vi "LV to ITX  Retrieve_SE mode.vi"(0 "File or Folder Path":path=path "B:/SketchSET/SA03008H.20180718/51-B+BG_0to15_0.25steps_@0-7T_1step_at.2Hz/SA03008H.20180718.000487.itx", 5 "offset":i32, 7 "length":i32=1, 9 "index":T2={"A"=3, "B"=5, "C"=3, "D"=5, "E"=3, "N1"=2, "N2"=2, "N3"=3, "N4"=4, "A 1"=8, "A 2"=10, "C 1"=5, "C 2"=1, "E 2"=4}, 11 "stop":bool, 12 "file contains 2D data?":bool) -> (1 "Spherical coordinates":dbl[][](array[numeric])=[[9.90056946810301, 45.0, 90.8270537879769]], 2 "long":cluster{i32[], dbl[]}(graph), 3 "G vs T":cluster{dbl[], dbl[]}(graph)={[7.00003046875], [0.0]}, 4 "A vs B":cluster{dbl[], dbl[]}[](graph), 6 "C vs D":cluster{dbl[], dbl[]}[](graph), 8 "E( = A)":dbl[][](graph)=[[0.010896697044372123], [0.010896697044372123], [0.010896697044372123], [0.010896697044372123], [0.010896697044372123], [0.010896697044372123], [0.010896697044372123], [0.010896697044372123], [0.010896697044372123], [0.010896697044372123], [0.010896697044372123], [0.010896697044372123], [0.010896697044372123], [0.010896697044372123], [0.010896697044372123], [0.010896697044372123], [0.010896697044372123], [0.010896697044372123], [0.010896697044372123], [0.010896697044372123], [0.010896697044372123], [0.010896697044372123], [0.010896697044372123], [0.010896697044372123], [0.010896697044372123], [0.010896697044372123], [0.010896697044372123], [0.010896697044372123], [0.010896697044372123], [0.010896697044372123], [0.010896697044372123], [0.010896697044372123], [0.010896697044372123], [0.010896697044372123], [0.010896697044372123], [0.010896697044372123], [0.010896697044372123], [0.010896697044372123], [0.010896697044372123], [0.010896697044372123], [0.010896697044372123], [0.010896697044372123], [0.010896697044372123], [0.010896697044372123], [0.010896697044372123], [0.010896697044372123], [0.010896697044372123], [0.010896697044372123], [0.010896697044372123], [0.010896697044372123], [0.010896697044372123], [0.010896697044372123], [0.010896697044372123], [0.010896697044372123], [0.010896697044372123], [0.010896697044372123], [0.010896697044372123], [0.010896697044372123], [0.010896697044372123], [0.010896697044372123], [0.010896697044372123], [0.010896697044372123], [0.010896697044372123], [0.010896697044372123], [0.010896697044372123], [0.010896697044372123], [0.010896697044372123], [0.010896697044372123], [0.010896697044372123], [0.010896697044372123], [0.010896697044372123], [0.010896697044372123], [0.010896697044372123], [0.010896697044372123], [0.010896697044372123], [0.010896697044372123], [0.010896697044372123], [0.010896697044372123], [0.010896697044372123], [0.010896697044372123], [0.010896697044372123], [0.010896697044372123], [0.010896697044372123], [0.010896697044372123], [0.010896697044372123], [0.010896697044372123], [0.010896697044372123], [0.010896697044372123], [0.010896697044372123], [0.010896697044372123], [0.010896697044372123], [0.010896697044372123], [0.010896697044372123], [0.010896697044372123], [0.010896697044372123], [0.010896697044372123], [0.010896697044372123], [0.010896697044372123], [0.010896697044372123], [0.010896697044372123], [0.010896697044372123], [0.010896697044372123], [0.010896697044372123], [0.010896697044372123], [0.010896697044372123], [0.010896697044372123], [0.010896697044372123], [0.010896697044372123], [0.010896697044372123], [0.010896697044372123], [0.010896697044372123], [0.010896697044372123], [0.010896697044372123], [0.010896697044372123], [0.010896697044372123], [0.010896697044372123], [0.010896697044372123], [0.010896697044372123], [0.010896697044372123], [0.010896697044372123], [0.010896697044372123], [0.010896697044372123], [0.010896697044372123], [0.010896697044372123], [0.010896697044372123], [0.010896697044372123], [0.010896697044372123], [0.010896697044372123], [0.010896697044372123], [0.010896697044372123], [0.010896697044372123], [0.010896697044372123], [0.010896697044372123], [0.010896697044372123], [0.010896697044372123], [0.010896697044372123], [0.010896697044372123], [0.010896697044372123], [0.010896697044372123], [0.010896697044372123], [0.010896697044372123], [0.010896697044372123], [0.010896697044372123], [0.010896697044372123], [0.010896697044372123], [0.010896697044372123], [0.010896697044372123], [0.010896697044372123], [0.010896697044372123], [0.010896697044372123], [0.010896697044372123], [0.010896697044372123], [0.010896697044372123], [0.010896697044372123], [0.010896697044372123], [0.010896697044372123], [0.010896697044372123], [0.010896697044372123], [0.010896697044372123], [0.010896697044372123], [0.010896697044372123], [0.010896697044372123], [0.010896697044372123], [0.010896697044372123], [0.010896697044372123], [0.010896697044372123], [0.010896697044372123], [0.010896697044372123], [0.010896697044372123], [0.010896697044372123], [0.010896697044372123], [0.010896697044372123], [0.010896697044372123], [0.010896697044372123], [0.010896697044372123], [0.010896697044372123], [0.010896697044372123], [0.010896697044372123], [0.010896697044372123], [0.010896697044372123], [0.010896697044372123], [0.010896697044372123], [0.010896697044372123], [0.010896697044372123], [0.010896697044372123], [0.010896697044372123], [0.010896697044372123], [0.010896697044372123], [0.010896697044372123], [0.010896697044372123], [0.010896697044372123], [0.010896697044372123], [0.010896697044372123], [0.010896697044372123], [0.010896697044372123], [0.010896697044372123], [0.010896697044372123], [0.010896697044372123], [0.010896697044372123], [0.010896697044372123], [0.010896697044372123], [0.010896697044372123], [0.010896697044372123], [0.010896697044372123], [0.010896697044372123], [0.010896697044372123], [0.010896697044372123], [0.010896697044372123], [0.010896697044372123], [0.010896697044372123], [0.010896697044372123], [0.010896697044372123], [0.010896697044372123], [0.010896697044372123], [0.010896697044372123], [0.010896697044372123], [0.010896697044372123], [0.010896697044372123], [0.010896697044372123], [0.010896697044372123], [0.010896697044372123], [0.010896697044372123], [0.010896697044372123], [0.010896697044372123], [0.010896697044372123], [0.010896697044372123], [0.010896697044372123], [0.010896697044372123], [0.010896697044372123], [0.010896697044372123], [0.010896697044372123], [0.010896697044372123], [0.010896697044372123], [0.010896697044372123], [0.010896697044372123], [0.010896697044372123], [0.010896697044372123], [0.010896697044372123], [0.010896697044372123], [0.010896697044372123], [0.010896697044372123], [0.010896697044372123], [0.010896697044372123], [0.010896697044372123], [0.010896697044372123], [0.010896697044372123], [0.010896697044372123], [0.010896697044372123], [0.010896697044372123], [0.010896697044372123], [0.010896697044372123], [0.010896697044372123], [0.010896697044372123], [0.010896697044372123], [0.010896697044372123], [0.010896697044372123], [0.010896697044372123], [0.010896697044372123], [0.010896697044372123], [0.010896697044372123], [0.010896697044372123], [0.010896697044372123], [0.010896697044372123], [0.010896697044372123], [0.010896697044372123], [0.010896697044372123], [0.010896697044372123], [0.010896697044372123], [0.010896697044372123], [0.010896697044372123], [0.010896697044372123], [0.010896697044372123], [0.010896697044372123], [0.010896697044372123], [0.010896697044372123], [0.010896697044372123], [0.010896697044372123], [0.010896697044372123], [0.010896697044372123], [0.010896697044372123], [0.010896697044372123], [0.010896697044372123], [0.010896697044372123], [0.010896697044372123], [0.010896697044372123], [0.010896697044372123], [0.010896697044372123], [0.010896697044372123], [0.010896697044372123], [0.010896697044372123], [0.010896697044372123], [0.010896697044372123], [0.010896697044372123], [0.010896697044372123], [0.010896697044372123], [0.010896697044372123], [0.010896697044372123], [0.010896697044372123], [0.010896697044372123], [0.010896697044372123], [0.010896697044372123], [0.010896697044372123], [0.010896697044372123], [0.010896697044372123], [0.010896697044372123], [0.010896697044372123], [0.010896697044372123], [0.010896697044372123], [0.010896697044372123], [0.010896697044372123], [0.010896697044372123], [0.010896697044372123], [0.010896697044372123], [0.010896697044372123], [0.010896697044372123], [0.010896697044372123], [0.010896697044372123], [0.010896697044372123], [0.010896697044372123], [0.010896697044372123], [0.010896697044372123], [0.010896697044372123], [0.010896697044372123], [0.010896697044372123], [0.010896697044372123], [0.010896697044372123], [0.010896697044372123], [0.010896697044372123], [0.010896697044372123], [0.010896697044372123], [0.010896697044372123], [0.010896697044372123], [0.010896697044372123], [0.010896697044372123], [0.010896697044372123], [0.010896697044372123], [0.010896697044372123], [0.010896697044372123], [0.010896697044372123], [0.010896697044372123], [0.010896697044372123], [0.010896697044372123], [0.010896697044372123], [0.010896697044372123], [0.010896697044372123], [0.010896697044372123], [0.010896697044372123], [0.010896697044372123], [0.010896697044372123], [0.010896697044372123], [0.010896697044372123], [0.010896697044372123], [0.010896697044372123], [0.010896697044372123], [0.010896697044372123], [0.010896697044372123], [0.010896697044372123], [0.010896697044372123], [0.010896697044372123], [0.010896697044372123], [0.010896697044372123], [0.010896697044372123], [0.010896697044372123], [0.010896697044372123], [0.010896697044372123], [0.010896697044372123], [0.010896697044372123], [0.010896697044372123], [0.010896697044372123], [0.010896697044372123], [0.010896697044372123], [0.010896697044372123], [0.010896697044372123], [0.010896697044372123], [0.010896697044372123], [0.010896697044372123], [0.010896697044372123], [0.010896697044372123], [0.010896697044372123], [0.010896697044372123], [0.010896697044372123], [0.010896697044372123], [0.010896697044372123], [0.010896697044372123], [0.010896697044372123], [0.010896697044372123], [0.010896697044372123], [0.010896697044372123], [0.010896697044372123], [0.010896697044372123], [0.010896697044372123], [0.010896697044372123], [0.010896697044372123], [0.010896697044372123], [0.010896697044372123], [0.010896697044372123], [0.010896697044372123], [0.010896697044372123], [0.010896697044372123], [0.010896697044372123], [0.010896697044372123], [0.010896697044372123], [0.010896697044372123], [0.010896697044372123], [0.010896697044372123], [0.010896697044372123], [0.010896697044372123], [0.010896697044372123], [0.010896697044372123], [0.010896697044372123], [0.010896697044372123], [0.010896697044372123], [0.010896697044372123], [0.010896697044372123], [0.010896697044372123], [0.010896697044372123], [0.010896697044372123], [0.010896697044372123], [0.010896697044372123], [0.010896697044372123], [0.010896697044372123], [0.010896697044372123], [0.010896697044372123], [0.010896697044372123], [0.010896697044372123], [0.010896697044372123], [0.010896697044372123], [0.010896697044372123], [0.010896697044372123], [0.010896697044372123], [0.010896697044372123], [0.010896697044372123], [0.010896697044372123], [0.010896697044372123], [0.010896697044372123], [0.010896697044372123], [0.010896697044372123], [0.010896697044372123], [0.010896697044372123], [0.010896697044372123], [0.010896697044372123], [0.010896697044372123], [0.010896697044372123], [0.010896697044372123], [0.010896697044372123], [0.010896697044372123], [0.010896697044372123], [0.010896697044372123], [0.010896697044372123], [0.010896697044372123], [0.010896697044372123], [0.010896697044372123], [0.010896697044372123], [0.010896697044372123], [0.010896697044372123], [0.010896697044372123], [0.010896697044372123], [0.010896697044372123], [0.010896697044372123], [0.010896697044372123], [0.010896697044372123], [0.010896697044372123], [0.010896697044372123], [0.010896697044372123], [0.010896697044372123], [0.010896697044372123], [0.010896697044372123], [0.010896697044372123], [0.010896697044372123], [0.010896697044372123], [0.010896697044372123], [0.010896697044372123], [0.010896697044372123], [0.010896697044372123], [0.010896697044372123], [0.010896697044372123], [0.010896697044372123], [0.010896697044372123], [0.010896697044372123], [0.010896697044372123], [0.010896697044372123], [0.010896697044372123], [0.010896697044372123], [0.010896697044372123], [0.010896697044372123], [0.010896697044372123], [0.010896697044372123], [0.010896697044372123], [0.010896697044372123], [0.010896697044372123], [0.010896697044372123], [0.010896697044372123], [0.010896697044372123], [0.010896697044372123], [0.010896697044372123], [0.010896697044372123], [0.010896697044372123], [0.010896697044372123], [0.010896697044372123], [0.010896697044372123], [0.010896697044372123], [0.010896697044372123], [0.010896697044372123], [0.010896697044372123], [0.010896697044372123], [0.010896697044372123], [0.010896697044372123], [0.010896697044372123], [0.010896697044372123], [0.010896697044372123], [0.010896697044372123], [0.010896697044372123], [0.010896697044372123], [0.010896697044372123], [0.010896697044372123], [0.010896697044372123], [0.010896697044372123], [0.010896697044372123], [0.010896697044372123], [0.010896697044372123], [0.010896697044372123], [0.010896697044372123], [0.010896697044372123], [0.010896697044372123], [0.010896697044372123], [0.010896697044372123], [0.010896697044372123], [0.010896697044372123], [0.010896697044372123], [0.010896697044372123], [0.010896697044372123], [0.010896697044372123], [0.010896697044372123], [0.010896697044372123], [0.010896697044372123], [0.010896697044372123], [0.010896697044372123], [0.010896697044372123], [0.010896697044372123], [0.010896697044372123], [0.010896697044372123], [0.010896697044372123], [0.010896697044372123], [0.010896697044372123], [0.010896697044372123], [0.010896697044372123], [0.010896697044372123], [0.010896697044372123], [0.010896697044372123], [0.010896697044372123], [0.010896697044372123], [0.010896697044372123], [0.010896697044372123], [0.010896697044372123], [0.010896697044372123], [0.010896697044372123], [0.010896697044372123], [0.010896697044372123], [0.010896697044372123], [0.010896697044372123], [0.010896697044372123], [0.010896697044372123], [0.010896697044372123], [0.010896697044372123], [0.010896697044372123], [0.010896697044372123], [0.010896697044372123], [0.010896697044372123], [0.010896697044372123], [0.010896697044372123], [0.010896697044372123], [0.010896697044372123], [0.010896697044372123], [0.010896697044372123], [0.010896697044372123], [0.010896697044372123], [0.010896697044372123], [0.010896697044372123], [0.010896697044372123], [0.010896697044372123], [0.010896697044372123], [0.010896697044372123], [0.010896697044372123], [0.010896697044372123], [0.010896697044372123], [0.010896697044372123], [0.010896697044372123], [0.010896697044372123], [0.010896697044372123], [0.010896697044372123], [0.010896697044372123], [0.010896697044372123], [0.010896697044372123], [0.010896697044372123], [0.010896697044372123], [0.010896697044372123], [0.010896697044372123], [0.010896697044372123], [0.010896697044372123], [0.010896697044372123], [0.010896697044372123], [0.010896697044372123], [0.010896697044372123], [0.010896697044372123], [0.010896697044372123], [0.010896697044372123], [0.010896697044372123], [0.010896697044372123], [0.010896697044372123], [0.010896697044372123], [0.010896697044372123], [0.010896697044372123], [0.010896697044372123], [0.010896697044372123], [0.010896697044372123], [0.010896697044372123], [0.010896697044372123], [0.010896697044372123], [0.010896697044372123], [0.010896697044372123], [0.010896697044372123], [0.010896697044372123], [0.010896697044372123], [0.010896697044372123], [0.010896697044372123], [0.010896697044372123], [0.010896697044372123], [0.010896697044372123], [0.010896697044372123], [0.010896697044372123], [0.010896697044372123], [0.010896697044372123], [0.010896697044372123], [0.010896697044372123], [0.010896697044372123], [0.010896697044372123], [0.010896697044372123], [0.010896697044372123], [0.010896697044372123], [0.010896697044372123], [0.010896697044372123], [0.010896697044372123], [0.010896697044372123], [0.010896697044372123], [0.010896697044372123], [0.010896697044372123], [0.010896697044372123], [0.010896697044372123], [0.010896697044372123], [0.010896697044372123], [0.010896697044372123], [0.010896697044372123], [0.010896697044372123], [0.010896697044372123], [0.010896697044372123], [0.010896697044372123], [0.010896697044372123], [0.010896697044372123], [0.010896697044372123], [0.010896697044372123], [0.010896697044372123], [0.010896697044372123], [0.010896697044372123], [0.010896697044372123], [0.010896697044372123], [0.010896697044372123], [0.010896697044372123], [0.010896697044372123], [0.010896697044372123], [0.010896697044372123], [0.010896697044372123], [0.010896697044372123], [0.010896697044372123], [0.010896697044372123], [0.010896697044372123], [0.010896697044372123], [0.010896697044372123], [0.010896697044372123], [0.010896697044372123], [0.010896697044372123], [0.010896697044372123], [0.010896697044372123], [0.010896697044372123], [0.010896697044372123], [0.010896697044372123], [0.010896697044372123], [0.010896697044372123], [0.010896697044372123], [0.010896697044372123], [0.010896697044372123], [0.010896697044372123], [0.010896697044372123], [0.010896697044372123], [0.010896697044372123], [0.010896697044372123], [0.010896697044372123], [0.010896697044372123], [0.010896697044372123], [0.010896697044372123], [0.010896697044372123], [0.010896697044372123], [0.010896697044372123], [0.010896697044372123], [0.010896697044372123], [0.010896697044372123], [0.010896697044372123], [0.010896697044372123], [0.010896697044372123], [0.010896697044372123], [0.010896697044372123], [0.010896697044372123], [0.010896697044372123], [0.010896697044372123], [0.010896697044372123], [0.010896697044372123], [0.010896697044372123], [0.010896697044372123], [0.010896697044372123], [0.010896697044372123], [0.010896697044372123], [0.010896697044372123], [0.010896697044372123], [0.010896697044372123], [0.010896697044372123], [0.010896697044372123], [0.010896697044372123], [0.010896697044372123], [0.010896697044372123], [0.010896697044372123], [0.010896697044372123], [0.010896697044372123], [0.010896697044372123], [0.010896697044372123], [0.010896697044372123], [0.010896697044372123], [0.010896697044372123], [0.010896697044372123], [0.010896697044372123], [0.010896697044372123], [0.010896697044372123], [0.010896697044372123], [0.010896697044372123], [0.010896697044372123], [0.010896697044372123], [0.010896697044372123], [0.010896697044372123], [0.010896697044372123], [0.010896697044372123], [0.010896697044372123], [0.010896697044372123], [0.010896697044372123], [0.010896697044372123], [0.010896697044372123], [0.010896697044372123], [0.010896697044372123], [0.010896697044372123], [0.010896697044372123], [0.010896697044372123], [0.010896697044372123], [0.010896697044372123], [0.010896697044372123], [0.010896697044372123], [0.010896697044372123], [0.010896697044372123], [0.010896697044372123], [0.010896697044372123], [0.010896697044372123], [0.010896697044372123], [0.010896697044372123], [0.010896697044372123], [0.010896697044372123], [0.010896697044372123], [0.010896697044372123], [0.010896697044372123], [0.010896697044372123], [0.010896697044372123], [0.010896697044372123], [0.010896697044372123], [0.010896697044372123], [0.010896697044372123], [0.010896697044372123], [0.010896697044372123], [0.010896697044372123], [0.010896697044372123], [0.010896697044372123], [0.010896697044372123], [0.010896697044372123], [0.010896697044372123], [0.010896697044372123], [0.010896697044372123], [0.010896697044372123], [0.010896697044372123], [0.010896697044372123], [0.010896697044372123], [0.010896697044372123], [0.010896697044372123], [0.010896697044372123], [0.010896697044372123], [0.010896697044372123], [0.010896697044372123], [0.010896697044372123], [0.010896697044372123], [0.010896697044372123], [0.010896697044372123], [0.010896697044372123], [0.010896697044372123], [0.010896697044372123], [0.010896697044372123], [0.010896697044372123], [0.010896697044372123], [0.010896697044372123], [0.010896697044372123], [0.010896697044372123], [0.010896697044372123], [0.010896697044372123], [0.010896697044372123], [0.010896697044372123], [0.010896697044372123], [0.010896697044372123], [0.010896697044372123], [0.010896697044372123], [0.010896697044372123], [0.010896697044372123], [0.010896697044372123], [0.010896697044372123], [0.010896697044372123], [0.010896697044372123], [0.010896697044372123], [0.010896697044372123], [0.010896697044372123], [0.010896697044372123], [0.010896697044372123], [0.010896697044372123], [0.010896697044372123], [0.010896697044372123], [0.010896697044372123], [0.010896697044372123], [0.010896697044372123], [0.010896697044372123], [0.010896697044372123], [0.010896697044372123], [0.010896697044372123], [0.010896697044372123], [0.010896697044372123], [0.010896697044372123], [0.010896697044372123], [0.010896697044372123], [0.010896697044372123], [0.010896697044372123], [0.010896697044372123], [0.010896697044372123], [0.010896697044372123], [0.010896697044372123], [0.010896697044372123], [0.010896697044372123], [0.010896697044372123], [0.010896697044372123], [0.010896697044372123], [0.010896697044372123], [0.010896697044372123], [0.010896697044372123], [0.010896697044372123], [0.010896697044372123], [0.010896697044372123], [0.010896697044372123], [0.010896697044372123], [0.010896697044372123], [0.010896697044372123], [0.010896697044372123], [0.010896697044372123], [0.010896697044372123], [0.010896697044372123], [0.010896697044372123], [0.010896697044372123], [0.010896697044372123], [0.010896697044372123], [0.010896697044372123], [0.010896697044372123], [0.010896697044372123], [0.010896697044372123], [0.010896697044372123], [0.010896697044372123], [0.010896697044372123], [0.010896697044372123], [0.010896697044372123], [0.010896697044372123], [0.010896697044372123], [0.010896697044372123], [0.010896697044372123], [0.010896697044372123], [0.010896697044372123], [0.010896697044372123], [0.010896697044372123], [0.010896697044372123], [0.010896697044372123], [0.010896697044372123], [0.010896697044372123], [0.010896697044372123], [0.010896697044372123], [0.010896697044372123], [0.010896697044372123], [0.010896697044372123], [0.010896697044372123], [0.010896697044372123], [0.010896697044372123], [0.010896697044372123], [0.010896697044372123], [0.010896697044372123], [0.010896697044372123], [0.010896697044372123], [0.010896697044372123], [0.010896697044372123], [0.010896697044372123], [0.010896697044372123], [0.010896697044372123], [0.010896697044372123], [0.010896697044372123], [0.010896697044372123], [0.010896697044372123], [0.010896697044372123], [0.010896697044372123], [0.010896697044372123], [0.010896697044372123], [0.010896697044372123], [0.010896697044372123], [0.010896697044372123], [0.010896697044372123], [0.010896697044372123], [0.010896697044372123], [0.010896697044372123], [0.010896697044372123], [0.010896697044372123], [0.010896697044372123], [0.010896697044372123], [0.010896697044372123], [0.010896697044372123], [0.010896697044372123], [0.010896697044372123], [0.010896697044372123], [0.010896697044372123], [0.010896697044372123], [0.010896697044372123], [0.010896697044372123], [0.010896697044372123], [0.010896697044372123], [0.010896697044372123], [0.010896697044372123], [0.010896697044372123], [0.010896697044372123], [0.010896697044372123], [0.010896697044372123], [0.010896697044372123], [0.010896697044372123], [0.010896697044372123], [0.010896697044372123], [0.010896697044372123], [0.010896697044372123], [0.010896697044372123], [0.010896697044372123], [0.010896697044372123], [0.010896697044372123], [0.010896697044372123], [0.010896697044372123], [0.010896697044372123], [0.010896697044372123], [0.010896697044372123], [0.010896697044372123], [0.010896697044372123], [0.010896697044372123], [0.010896697044372123], [0.010896697044372123], [0.010896697044372123], [0.010896697044372123], [0.010896697044372123], [0.010896697044372123], [0.010896697044372123], [0.010896697044372123], [0.010896697044372123], [0.010896697044372123], [0.010896697044372123], [0.010896697044372123], [0.010896697044372123], [0.010896697044372123], [0.010896697044372123], [0.010896697044372123], [0.010896697044372123], [0.010896697044372123], [0.010896697044372123], [0.010896697044372123], [0.010896697044372123], [0.010896697044372123], [0.010896697044372123], [0.010896697044372123], [0.010896697044372123], [0.010896697044372123], [0.010896697044372123], [0.010896697044372123], [0.010896697044372123], [0.010896697044372123], [0.010896697044372123], [0.010896697044372123], [0.010896697044372123], [0.010896697044372123], [0.010896697044372123], [0.010896697044372123], [0.010896697044372123], [0.010896697044372123], [0.010896697044372123], [0.010896697044372123], [0.010896697044372123], [0.010896697044372123], [0.010896697044372123], [0.010896697044372123], [0.010896697044372123], [0.010896697044372123], [0.010896697044372123], [0.010896697044372123], [0.010896697044372123], [0.010896697044372123], [0.010896697044372123], [0.010896697044372123], [0.010896697044372123], [0.010896697044372123], [0.010896697044372123], [0.010896697044372123], [0.010896697044372123], [0.010896697044372123], [0.010896697044372123], [0.010896697044372123], [0.010896697044372123], [0.010896697044372123], [0.010896697044372123], [0.010896697044372123], [0.010896697044372123], [0.010896697044372123], [0.010896697044372123], [0.010896697044372123], [0.010896697044372123], [0.010896697044372123], [0.010896697044372123], [0.010896697044372123], [0.010896697044372123], [0.010896697044372123], [0.010896697044372123], [0.010896697044372123], [0.010896697044372123], [0.010896697044372123], [0.010896697044372123], [0.010896697044372123], [0.010896697044372123], [0.010896697044372123], [0.010896697044372123], [0.010896697044372123], [0.010896697044372123], [0.010896697044372123], [0.010896697044372123], [0.010896697044372123], [0.010896697044372123], [0.010896697044372123], [0.010896697044372123], [0.010896697044372123], [0.010896697044372123], [0.010896697044372123], [0.010896697044372123], [0.010896697044372123], [0.010896697044372123], [0.010896697044372123], [0.010896697044372123], [0.010896697044372123], [0.010896697044372123], [0.010896697044372123], [0.010896697044372123], [0.010896697044372123], [0.010896697044372123], [0.010896697044372123], [0.010896697044372123], [0.010896697044372123], [0.010896697044372123], [0.010896697044372123], [0.010896697044372123], [0.010896697044372123], [0.010896697044372123], [0.010896697044372123], [0.010896697044372123], [0.010896697044372123], [0.010896697044372123], [0.010896697044372123], [0.010896697044372123], [0.010896697044372123], [0.010896697044372123], [0.010896697044372123], [0.010896697044372123], [0.010896697044372123], [0.010896697044372123], [0.010896697044372123], [0.010896697044372123], [0.010896697044372123], [0.010896697044372123], [0.010896697044372123], [0.010896697044372123], [0.010896697044372123], [0.010896697044372123], [0.010896697044372123], [0.010896697044372123], [0.010896697044372123], [0.010896697044372123], [0.010896697044372123], [0.010896697044372123], [0.010896697044372123], [0.010896697044372123], [0.010896697044372123], [0.010896697044372123], [0.010896697044372123], [0.010896697044372123], [0.010896697044372123], [0.010896697044372123], [0.010896697044372123], [0.010896697044372123], [0.010896697044372123], [0.010896697044372123], [0.010896697044372123], [0.010896697044372123], [0.010896697044372123], [0.010896697044372123], [0.010896697044372123], [0.010896697044372123], [0.010896697044372123], [0.010896697044372123], [0.010896697044372123], [0.010896697044372123], [0.010896697044372123], [0.010896697044372123], [0.010896697044372123], [0.010896697044372123], [0.010896697044372123], [0.010896697044372123], [0.010896697044372123], [0.010896697044372123], [0.010896697044372123], [0.010896697044372123], [0.010896697044372123], [0.010896697044372123], [0.010896697044372123], [0.010896697044372123], [0.010896697044372123], [0.010896697044372123], [0.010896697044372123], [0.010896697044372123], [0.010896697044372123], [0.010896697044372123], [0.010896697044372123], [0.010896697044372123], [0.010896697044372123], [0.010896697044372123], [0.010896697044372123], [0.010896697044372123], [0.010896697044372123], [0.010896697044372123], [0.010896697044372123], [0.010896697044372123], [0.010896697044372123], [0.010896697044372123], [0.010896697044372123], [0.010896697044372123], [0.010896697044372123], [0.010896697044372123], [0.010896697044372123], [0.010896697044372123], [0.010896697044372123], [0.010896697044372123], [0.010896697044372123], [0.010896697044372123], [0.010896697044372123], [0.010896697044372123], [0.010896697044372123], [0.010896697044372123], [0.010896697044372123], [0.010896697044372123], [0.010896697044372123], [0.010896697044372123], [0.010896697044372123], [0.010896697044372123], [0.010896697044372123], [0.010896697044372123], [0.010896697044372123], [0.010896697044372123], [0.010896697044372123], [0.010896697044372123], [0.010896697044372123], [0.010896697044372123], [0.010896697044372123], [0.010896697044372123], [0.010896697044372123], [0.010896697044372123], [0.010896697044372123], [0.010896697044372123], [0.010896697044372123], [0.010896697044372123], [0.010896697044372123], [0.010896697044372123], [0.010896697044372123], [0.010896697044372123], [0.010896697044372123], [0.010896697044372123], [0.010896697044372123], [0.010896697044372123], [0.010896697044372123], [0.010896697044372123], [0.010896697044372123], [0.010896697044372123], [0.010896697044372123], [0.010896697044372123], [0.010896697044372123], [0.010896697044372123], [0.010896697044372123], [0.010896697044372123], [0.010896697044372123], [0.010896697044372123], [0.010896697044372123], [0.010896697044372123], [0.010896697044372123], [0.010896697044372123], [0.010896697044372123], [0.010896697044372123], [0.010896697044372123], [0.010896697044372123], [0.010896697044372123], [0.010896697044372123], [0.010896697044372123], [0.010896697044372123], [0.010896697044372123], [0.010896697044372123], [0.010896697044372123], [0.010896697044372123], [0.010896697044372123], [0.010896697044372123], [0.010896697044372123], [0.010896697044372123], [0.010896697044372123], [0.010896697044372123], [0.010896697044372123], [0.010896697044372123], [0.010896697044372123], [0.010896697044372123], [0.010896697044372123], [0.010896697044372123], [0.010896697044372123], [0.010896697044372123], [0.010896697044372123], [0.010896697044372123], [0.010896697044372123], [0.010896697044372123], [0.010896697044372123], [0.010896697044372123], [0.010896697044372123], [0.010896697044372123], [0.010896697044372123], [0.010896697044372123], [0.010896697044372123], [0.010896697044372123], [0.010896697044372123], [0.010896697044372123], [0.010896697044372123], [0.010896697044372123], [0.010896697044372123], [0.010896697044372123], [0.010896697044372123], [0.010896697044372123], [0.010896697044372123], [0.010896697044372123], [0.010896697044372123], [0.010896697044372123], [0.010896697044372123], [0.010896697044372123], [0.010896697044372123], [0.010896697044372123], [0.010896697044372123], [0.010896697044372123], [0.010896697044372123], [0.010896697044372123], [0.010896697044372123], [0.010896697044372123], [0.010896697044372123], [0.010896697044372123], [0.010896697044372123], [0.010896697044372123], [0.010896697044372123], [0.010896697044372123], [0.010896697044372123], [0.010896697044372123], [0.010896697044372123], [0.010896697044372123], [0.010896697044372123], [0.010896697044372123], [0.010896697044372123], [0.010896697044372123], [0.010896697044372123], [0.010896697044372123], [0.010896697044372123], [0.010896697044372123], [0.010896697044372123], [0.010896697044372123], [0.010896697044372123], [0.010896697044372123], [0.010896697044372123], [0.010896697044372123], [0.010896697044372123], [0.010896697044372123], [0.010896697044372123], [0.010896697044372123], [0.010896697044372123], [0.010896697044372123], [0.010896697044372123], [0.010896697044372123], [0.010896697044372123], [0.010896697044372123], [0.010896697044372123], [0.010896697044372123], [0.010896697044372123], [0.010896697044372123], [0.010896697044372123], [0.010896697044372123], [0.010896697044372123], [0.010896697044372123], [0.010896697044372123], [0.010896697044372123], [0.010896697044372123], [0.010896697044372123], [0.010896697044372123], [0.010896697044372123], [0.010896697044372123], [0.010896697044372123], [0.010896697044372123], [0.010896697044372123], [0.010896697044372123], [0.010896697044372123], [0.010896697044372123], [0.010896697044372123], [0.010896697044372123], [0.010896697044372123], [0.010896697044372123], [0.010896697044372123], [0.010896697044372123], [0.010896697044372123], [0.010896697044372123], [0.010896697044372123], [0.010896697044372123], [0.010896697044372123], [0.010896697044372123], [0.010896697044372123], [0.010896697044372123], [0.010896697044372123], [0.010896697044372123], [0.010896697044372123], [0.010896697044372123], [0.010896697044372123], [0.010896697044372123], [0.010896697044372123], [0.010896697044372123], [0.010896697044372123], [0.010896697044372123], [0.010896697044372123], [0.010896697044372123], [0.010896697044372123], [0.010896697044372123], [0.010896697044372123], [0.010896697044372123], [0.010896697044372123], [0.010896697044372123], [0.010896697044372123], [0.010896697044372123], [0.010896697044372123], [0.010896697044372123], [0.010896697044372123], [0.010896697044372123], [0.010896697044372123], [0.010896697044372123], [0.010896697044372123], [0.010896697044372123], [0.010896697044372123], [0.010896697044372123], [0.010896697044372123], [0.010896697044372123], [0.010896697044372123], [0.010896697044372123], [0.010896697044372123], [0.010896697044372123], [0.010896697044372123], [0.010896697044372123], [0.010896697044372123], [0.010896697044372123], [0.010896697044372123], [0.010896697044372123], [0.010896697044372123], [0.010896697044372123], [0.010896697044372123], [0.010896697044372123], [0.010896697044372123], [0.010896697044372123], [0.010896697044372123], [0.010896697044372123], [0.010896697044372123], [0.010896697044372123], [0.010896697044372123], [0.010896697044372123], [0.010896697044372123], [0.010896697044372123], [0.010896697044372123], [0.010896697044372123], [0.010896697044372123], [0.010896697044372123], [0.010896697044372123], [0.010896697044372123], [0.010896697044372123], [0.010896697044372123], [0.010896697044372123], [0.010896697044372123], [0.010896697044372123], [0.010896697044372123], [0.010896697044372123], [0.010896697044372123], [0.010896697044372123], [0.010896697044372123], [0.010896697044372123], [0.010896697044372123], [0.010896697044372123], [0.010896697044372123], [0.010896697044372123], [0.010896697044372123], [0.010896697044372123], [0.010896697044372123], [0.010896697044372123], [0.010896697044372123], [0.010896697044372123], [0.010896697044372123], [0.010896697044372123], [0.010896697044372123], [0.010896697044372123], [0.010896697044372123], [0.010896697044372123], [0.010896697044372123], [0.010896697044372123], [0.010896697044372123], [0.010896697044372123], [0.010896697044372123], [0.010896697044372123], [0.010896697044372123], [0.010896697044372123], [0.010896697044372123], [0.010896697044372123], [0.010896697044372123], [0.010896697044372123], [0.010896697044372123], [0.010896697044372123], [0.010896697044372123], [0.010896697044372123], [0.010896697044372123], [0.010896697044372123], [0.010896697044372123], [0.010896697044372123], [0.010896697044372123], [0.010896697044372123], [0.010896697044372123], [0.010896697044372123], [0.010896697044372123], [0.010896697044372123], [0.010896697044372123], [0.010896697044372123], [0.010896697044372123], [0.010896697044372123], [0.010896697044372123], [0.010896697044372123], [0.010896697044372123], [0.010896697044372123], [0.010896697044372123], [0.010896697044372123], [0.010896697044372123], [0.010896697044372123], [0.010896697044372123], [0.010896697044372123], [0.010896697044372123], [0.010896697044372123], [0.010896697044372123], [0.010896697044372123], [0.010896697044372123], [0.010896697044372123], [0.010896697044372123], [0.010896697044372123], [0.010896697044372123], [0.010896697044372123], [0.010896697044372123], [0.010896697044372123], [0.010896697044372123], [0.010896697044372123], [0.010896697044372123], [0.010896697044372123], [0.010896697044372123], [0.010896697044372123], [0.010896697044372123], [0.010896697044372123], [0.010896697044372123], [0.010896697044372123], [0.010896697044372123], [0.010896697044372123], [0.010896697044372123], [0.010896697044372123], [0.010896697044372123], [0.010896697044372123], [0.010896697044372123], [0.010896697044372123], [0.010896697044372123], [0.010896697044372123], [0.010896697044372123], [0.010896697044372123], [0.010896697044372123], [0.010896697044372123], [0.010896697044372123], [0.010896697044372123], [0.010896697044372123], [0.010896697044372123], [0.010896697044372123], [0.010896697044372123], [0.010896697044372123], [0.010896697044372123], [0.010896697044372123], [0.010896697044372123], [0.010896697044372123], [0.010896697044372123], [0.010896697044372123], [0.010896697044372123], [0.010896697044372123], [0.010896697044372123], [0.010896697044372123], [0.010896697044372123], [0.010896697044372123], [0.010896697044372123], [0.010896697044372123], [0.010896697044372123], [0.010896697044372123], [0.010896697044372123], [0.010896697044372123], [0.010896697044372123], [0.010896697044372123], [0.010896697044372123], [0.010896697044372123], [0.010896697044372123], [0.010896697044372123], [0.010896697044372123], [0.010896697044372123], [0.010896697044372123], [0.010896697044372123], [0.010896697044372123], [0.010896697044372123], [0.010896697044372123], [0.010896697044372123], [0.010896697044372123], [0.010896697044372123], [0.010896697044372123], [0.010896697044372123], [0.010896697044372123], [0.010896697044372123], [0.010896697044372123], [0.010896697044372123], [0.010896697044372123], [0.010896697044372123], [0.010896697044372123], [0.010896697044372123], [0.010896697044372123], [0.010896697044372123], [0.010896697044372123], [0.010896697044372123], [0.010896697044372123], [0.010896697044372123], [0.010896697044372123], [0.010896697044372123], [0.010896697044372123], [0.010896697044372123], [0.010896697044372123], [0.010896697044372123], [0.010896697044372123], [0.010896697044372123], [0.010896697044372123], [0.010896697044372123], [0.010896697044372123], [0.010896697044372123], [0.010896697044372123], [0.010896697044372123], [0.010896697044372123], [0.010896697044372123], [0.010896697044372123], [0.010896697044372123], [0.010896697044372123], [0.010896697044372123], [0.010896697044372123], [0.010896697044372123], [0.010896697044372123], [0.010896697044372123], [0.010896697044372123], [0.010896697044372123], [0.010896697044372123], [0.010896697044372123], [0.010896697044372123], [0.010896697044372123], [0.010896697044372123], [0.010896697044372123], [0.010896697044372123], [0.010896697044372123], [0.010896697044372123], [0.010896697044372123], [0.010896697044372123], [0.010896697044372123], [0.010896697044372123], [0.010896697044372123], [0.010896697044372123], [0.010896697044372123], [0.010896697044372123], [0.010896697044372123], [0.010896697044372123], [0.010896697044372123], [0.010896697044372123], [0.010896697044372123], [0.010896697044372123], [0.010896697044372123], [0.010896697044372123], [0.010896697044372123], [0.010896697044372123], [0.010896697044372123], [0.010896697044372123], [0.010896697044372123], [0.010896697044372123], [0.010896697044372123], [0.010896697044372123], [0.010896697044372123], [0.010896697044372123], [0.010896697044372123], [0.010896697044372123], [0.010896697044372123], [0.010896697044372123], [0.010896697044372123], [0.010896697044372123], [0.010896697044372123], [0.010896697044372123], [0.010896697044372123], [0.010896697044372123], [0.010896697044372123], [0.010896697044372123], [0.010896697044372123], [0.010896697044372123], [0.010896697044372123], [0.010896697044372123], [0.010896697044372123], [0.010896697044372123], [0.010896697044372123], [0.010896697044372123], [0.010896697044372123], [0.010896697044372123], [0.010896697044372123], [0.010896697044372123], [0.010896697044372123], [0.010896697044372123], [0.010896697044372123], [0.010896697044372123], [0.010896697044372123], [0.010896697044372123], [0.010896697044372123], [0.010896697044372123], [0.010896697044372123], [0.010896697044372123], [0.010896697044372123], [0.010896697044372123], [0.010896697044372123], [0.010896697044372123], [0.010896697044372123], [0.010896697044372123], [0.010896697044372123], [0.010896697044372123], [0.010896697044372123], [0.010896697044372123], [0.010896697044372123], [0.010896697044372123], [0.010896697044372123], [0.010896697044372123], [0.010896697044372123], [0.010896697044372123], [0.010896697044372123], [0.010896697044372123], [0.010896697044372123], [0.010896697044372123], [0.010896697044372123], [0.010896697044372123], [0.010896697044372123], [0.010896697044372123], [0.010896697044372123], [0.010896697044372123], [0.010896697044372123], [0.010896697044372123], [0.010896697044372123], [0.010896697044372123], [0.010896697044372123], [0.010896697044372123], [0.010896697044372123], [0.010896697044372123], [0.010896697044372123], [0.010896697044372123], [0.010896697044372123], [0.010896697044372123], [0.010896697044372123], [0.010896697044372123], [0.010896697044372123], [0.010896697044372123], [0.010896697044372123], [0.010896697044372123], [0.010896697044372123], [0.010896697044372123], [0.010896697044372123], [0.010896697044372123], [0.010896697044372123], [0.010896697044372123], [0.010896697044372123], [0.010896697044372123], [0.010896697044372123], [0.010896697044372123], [0.010896697044372123], [0.010896697044372123], [0.010896697044372123], [0.010896697044372123], [0.010896697044372123], [0.010896697044372123], [0.010896697044372123], [0.010896697044372123], [0.010896697044372123], [0.010896697044372123], [0.010896697044372123], [0.010896697044372123], [0.010896697044372123], [0.010896697044372123], [0.010896697044372123], [0.010896697044372123], [0.010896697044372123], [0.010896697044372123], [0.010896697044372123], [0.010896697044372123], [0.010896697044372123], [0.010896697044372123], [0.010896697044372123], [0.010896697044372123], [0.010896697044372123], [0.010896697044372123], [0.010896697044372123], [0.010896697044372123], [0.010896697044372123], [0.010896697044372123], [0.010896697044372123], [0.010896697044372123], [0.010896697044372123], [0.010896697044372123], [0.010896697044372123], [0.010896697044372123], [0.010896697044372123], [0.010896697044372123], [0.010896697044372123], [0.010896697044372123], [0.010896697044372123], [0.010896697044372123], [0.010896697044372123], [0.010896697044372123], [0.010896697044372123], [0.010896697044372123], [0.010896697044372123], [0.010896697044372123], [0.010896697044372123], [0.010896697044372123], [0.010896697044372123], [0.010896697044372123], [0.010896697044372123], [0.010896697044372123], [0.010896697044372123], [0.010896697044372123], [0.010896697044372123], [0.010896697044372123], [0.010896697044372123], [0.010896697044372123], [0.010896697044372123], [0.010896697044372123], [0.010896697044372123], [0.010896697044372123], [0.010896697044372123], [0.010896697044372123], [0.010896697044372123], [0.010896697044372123], [0.010896697044372123], [0.010896697044372123], [0.010896697044372123], [0.010896697044372123], [0.010896697044372123], [0.010896697044372123], [0.010896697044372123], [0.010896697044372123], [0.010896697044372123], [0.010896697044372123], [0.010896697044372123], [0.010896697044372123], [0.010896697044372123], [0.010896697044372123], [0.010896697044372123], [0.010896697044372123], [0.010896697044372123], [0.010896697044372123], [0.010896697044372123], [0.010896697044372123], [0.010896697044372123], [0.010896697044372123], [0.010896697044372123], [0.010896697044372123], [0.010896697044372123], [0.010896697044372123], [0.010896697044372123], [0.010896697044372123], [0.010896697044372123], [0.010896697044372123], [0.010896697044372123], [0.010896697044372123], [0.010896697044372123], [0.010896697044372123], [0.010896697044372123], [0.010896697044372123], [0.010896697044372123], [0.010896697044372123], [0.010896697044372123], [0.010896697044372123], [0.010896697044372123], [0.010896697044372123], [0.010896697044372123], [0.010896697044372123], [0.010896697044372123], [0.010896697044372123], [0.010896697044372123], [0.010896697044372123], [0.010896697044372123], [0.010896697044372123], [0.010896697044372123], [0.010896697044372123], [0.010896697044372123], [0.010896697044372123], [0.010896697044372123], [0.010896697044372123], [0.010896697044372123], [0.010896697044372123], [0.010896697044372123], [0.010896697044372123], [0.010896697044372123], [0.010896697044372123], [0.010896697044372123], [0.010896697044372123], [0.010896697044372123], [0.010896697044372123], [0.010896697044372123], [0.010896697044372123], [0.010896697044372123], [0.010896697044372123], [0.010896697044372123], [0.010896697044372123], [0.010896697044372123], [0.010896697044372123], [0.010896697044372123], [0.010896697044372123], [0.010896697044372123], [0.010896697044372123], [0.010896697044372123], [0.010896697044372123], [0.010896697044372123], [0.010896697044372123], [0.010896697044372123], [0.010896697044372123], [0.010896697044372123], [0.010896697044372123], [0.010896697044372123], [0.010896697044372123], [0.010896697044372123], [0.010896697044372123], [0.010896697044372123], [0.010896697044372123], [0.010896697044372123], [0.010896697044372123], [0.010896697044372123], [0.010896697044372123], [0.010896697044372123], [0.010896697044372123], [0.010896697044372123], [0.010896697044372123], [0.010896697044372123], [0.010896697044372123], [0.010896697044372123], [0.010896697044372123], [0.010896697044372123], [0.010896697044372123], [0.010896697044372123], [0.010896697044372123], [0.010896697044372123], [0.010896697044372123], [0.010896697044372123], [0.010896697044372123], [0.010896697044372123], [0.010896697044372123], [0.010896697044372123], [0.010896697044372123], [0.010896697044372123], [0.010896697044372123], [0.010896697044372123], [0.010896697044372123], [0.010896697044372123], [0.010896697044372123], [0.010896697044372123], [0.010896697044372123], [0.010896697044372123], [0.010896697044372123], [0.010896697044372123], [0.010896697044372123], [0.010896697044372123], [0.010896697044372123], [0.010896697044372123], [0.010896697044372123], [0.010896697044372123], [0.010896697044372123], [0.010896697044372123], [0.010896697044372123], [0.010896697044372123], [0.010896697044372123], [0.010896697044372123], [0.010896697044372123], [0.010896697044372123], [0.010896697044372123], [0.010896697044372123], [0.010896697044372123], [0.010896697044372123], [0.010896697044372123], [0.010896697044372123], [0.010896697044372123], [0.010896697044372123], [0.010896697044372123], [0.010896697044372123], [0.010896697044372123], [0.010896697044372123], [0.010896697044372123], [0.010896697044372123], [0.010896697044372123], [0.010896697044372123], [0.010896697044372123], [0.010896697044372123], [0.010896697044372123], [0.010896697044372123], [0.010896697044372123], [0.010896697044372123], [0.010896697044372123], [0.010896697044372123], [0.010896697044372123], [0.010896697044372123], [0.010896697044372123], [0.010896697044372123], [0.010896697044372123], [0.010896697044372123], [0.010896697044372123], [0.010896697044372123], [0.010896697044372123], [0.010896697044372123], [0.010896697044372123], [0.010896697044372123], [0.010896697044372123], [0.010896697044372123], [0.010896697044372123], [0.010896697044372123], [0.010896697044372123], [0.010896697044372123], [0.010896697044372123], [0.010896697044372123], [0.010896697044372123], [0.010896697044372123], [0.010896697044372123], [0.010896697044372123], [0.010896697044372123], [0.010896697044372123], [0.010896697044372123], [0.010896697044372123], [0.010896697044372123], [0.010896697044372123], [0.010896697044372123], [0.010896697044372123], [0.010896697044372123], [0.010896697044372123], [0.010896697044372123], [0.010896697044372123], [0.010896697044372123], [0.010896697044372123], [0.010896697044372123], [0.010896697044372123], [0.010896697044372123], [0.010896697044372123], [0.010896697044372123], [0.010896697044372123], [0.010896697044372123], [0.010896697044372123], [0.010896697044372123], [0.010896697044372123], [0.010896697044372123], [0.010896697044372123], [0.010896697044372123], [0.010896697044372123], [0.010896697044372123], [0.010896697044372123], [0.010896697044372123], [0.010896697044372123], [0.010896697044372123], [0.010896697044372123], [0.010896697044372123], [0.010896697044372123], [0.010896697044372123], [0.010896697044372123], [0.010896697044372123], [0.010896697044372123], [0.010896697044372123], [0.010896697044372123], [0.010896697044372123], [0.010896697044372123], [0.010896697044372123], [0.010896697044372123], [0.010896697044372123], [0.010896697044372123], [0.010896697044372123], [0.010896697044372123], [0.010896697044372123], [0.010896697044372123], [0.010896697044372123], [0.010896697044372123], [0.010896697044372123], [0.010896697044372123], [0.010896697044372123], [0.010896697044372123], [0.010896697044372123], [0.010896697044372123], [0.010896697044372123], [0.010896697044372123], [0.010896697044372123], [0.010896697044372123], [0.010896697044372123], [0.010896697044372123], [0.010896697044372123], [0.010896697044372123], [0.010896697044372123], [0.010896697044372123], [0.010896697044372123], [0.010896697044372123], [0.010896697044372123], [0.010896697044372123], [0.010896697044372123], [0.010896697044372123], [0.010896697044372123], [0.010896697044372123], [0.010896697044372123], [0.010896697044372123], [0.010896697044372123], [0.010896697044372123], [0.010896697044372123], [0.010896697044372123], [0.010896697044372123], [0.010896697044372123], [0.010896697044372123], [0.010896697044372123], [0.010896697044372123], [0.010896697044372123], [0.010896697044372123], [0.010896697044372123], [0.010896697044372123], [0.010896697044372123], [0.010896697044372123], [0.010896697044372123], [0.010896697044372123], [0.010896697044372123], [0.010896697044372123], [0.010896697044372123], [0.010896697044372123], [0.010896697044372123], [0.010896697044372123], [0.010896697044372123], [0.010896697044372123], [0.010896697044372123], [0.010896697044372123], [0.010896697044372123], [0.010896697044372123], [0.010896697044372123], [0.010896697044372123], [0.010896697044372123], [0.010896697044372123], [0.010896697044372123], [0.010896697044372123], [0.010896697044372123], [0.010896697044372123], [0.010896697044372123], [0.010896697044372123], [0.010896697044372123], [0.010896697044372123], [0.010896697044372123], [0.010896697044372123], [0.010896697044372123], [0.010896697044372123], [0.010896697044372123], [0.010896697044372123], [0.010896697044372123], [0.010896697044372123], [0.010896697044372123], [0.010896697044372123], [0.010896697044372123], [0.010896697044372123], [0.010896697044372123], [0.010896697044372123], [0.010896697044372123], [0.010896697044372123], [0.010896697044372123], [0.010896697044372123], [0.010896697044372123], [0.010896697044372123], [0.010896697044372123], [0.010896697044372123], [0.010896697044372123], [0.010896697044372123], [0.010896697044372123], [0.010896697044372123], [0.010896697044372123], [0.010896697044372123], [0.010896697044372123], [0.010896697044372123], [0.010896697044372123], [0.010896697044372123], [0.010896697044372123], [0.010896697044372123], [0.010896697044372123], [0.010896697044372123], [0.010896697044372123], [0.010896697044372123], [0.010896697044372123], [0.010896697044372123], [0.010896697044372123], [0.010896697044372123], [0.010896697044372123], [0.010896697044372123], [0.010896697044372123], [0.010896697044372123], [0.010896697044372123], [0.010896697044372123], [0.010896697044372123], [0.010896697044372123], [0.010896697044372123], [0.010896697044372123], [0.010896697044372123], [0.010896697044372123], [0.010896697044372123], [0.010896697044372123], [0.010896697044372123], [0.010896697044372123], [0.010896697044372123], [0.010896697044372123], [0.010896697044372123], [0.010896697044372123], [0.010896697044372123], [0.010896697044372123], [0.010896697044372123], [0.010896697044372123], [0.010896697044372123], [0.010896697044372123], [0.010896697044372123], [0.010896697044372123], [0.010896697044372123], [0.010896697044372123], [0.010896697044372123], [0.010896697044372123], [0.010896697044372123], [0.010896697044372123], [0.010896697044372123], [0.010896697044372123], [0.010896697044372123], [0.010896697044372123], [0.010896697044372123], [0.010896697044372123], [0.010896697044372123], [0.010896697044372123], [0.010896697044372123], [0.010896697044372123], [0.010896697044372123], [0.010896697044372123], [0.010896697044372123], [0.010896697044372123], [0.010896697044372123], [0.010896697044372123], [0.010896697044372123], [0.010896697044372123], [0.010896697044372123], [0.010896697044372123], [0.010896697044372123], [0.010896697044372123], [0.010896697044372123], [0.010896697044372123], [0.010896697044372123], [0.010896697044372123], [0.010896697044372123], [0.010896697044372123], [0.010896697044372123], [0.010896697044372123], [0.010896697044372123], [0.010896697044372123], [0.010896697044372123], [0.010896697044372123], [0.010896697044372123], [0.010896697044372123], [0.010896697044372123], [0.010896697044372123], [0.010896697044372123], [0.010896697044372123], [0.010896697044372123], [0.010896697044372123], [0.010896697044372123], [0.010896697044372123], [0.010896697044372123], [0.010896697044372123], [0.010896697044372123], [0.010896697044372123], [0.010896697044372123], [0.010896697044372123], [0.010896697044372123], [0.010896697044372123], [0.010896697044372123], [0.010896697044372123], [0.010896697044372123], [0.010896697044372123], [0.010896697044372123], [0.010896697044372123], [0.010896697044372123], [0.010896697044372123], [0.010896697044372123], [0.010896697044372123], [0.010896697044372123], [0.010896697044372123], [0.010896697044372123], [0.010896697044372123], [0.010896697044372123], [0.010896697044372123], [0.010896697044372123], [0.010896697044372123], [0.010896697044372123], [0.010896697044372123], [0.010896697044372123], [0.010896697044372123], [0.010896697044372123], [0.010896697044372123], [0.010896697044372123], [0.010896697044372123], [0.010896697044372123], [0.010896697044372123], [0.010896697044372123], [0.010896697044372123], [0.010896697044372123], [0.010896697044372123], [0.010896697044372123], [0.010896697044372123], [0.010896697044372123], [0.010896697044372123], [0.010896697044372123], [0.010896697044372123], [0.010896697044372123], [0.010896697044372123], [0.010896697044372123], [0.010896697044372123], [0.010896697044372123], [0.010896697044372123], [0.010896697044372123], [0.010896697044372123], [0.010896697044372123], [0.010896697044372123], [0.010896697044372123], [0.010896697044372123], [0.010896697044372123], [0.010896697044372123], [0.010896697044372123], [0.010896697044372123], [0.010896697044372123], [0.010896697044372123], [0.010896697044372123], [0.010896697044372123], [0.010896697044372123], [0.010896697044372123], [0.010896697044372123], [0.010896697044372123], [0.010896697044372123], [0.010896697044372123], [0.010896697044372123], [0.010896697044372123], [0.010896697044372123], [0.010896697044372123], [0.010896697044372123], [0.010896697044372123], [0.010896697044372123], [0.010896697044372123], [0.010896697044372123], [0.010896697044372123], [0.010896697044372123], [0.010896697044372123], [0.010896697044372123], [0.010896697044372123], [0.010896697044372123], [0.010896697044372123], [0.010896697044372123], [0.010896697044372123], [0.010896697044372123], [0.010896697044372123], [0.010896697044372123], [0.010896697044372123], [0.010896697044372123], [0.010896697044372123], [0.010896697044372123], [0.010896697044372123], [0.010896697044372123], [0.010896697044372123], [0.010896697044372123], [0.010896697044372123], [0.010896697044372123], [0.010896697044372123], [0.010896697044372123], [0.010896697044372123], [0.010896697044372123], [0.010896697044372123], [0.010896697044372123], [0.010896697044372123], [0.010896697044372123], [0.010896697044372123], [0.010896697044372123], [0.010896697044372123], [0.010896697044372123], [0.010896697044372123], [0.010896697044372123], [0.010896697044372123], [0.010896697044372123], [0.010896697044372123], [0.010896697044372123], [0.010896697044372123], [0.010896697044372123], [0.010896697044372123], [0.010896697044372123], [0.010896697044372123], [0.010896697044372123], [0.010896697044372123], [0.010896697044372123], [0.010896697044372123], [0.010896697044372123], [0.010896697044372123], [0.010896697044372123], [0.010896697044372123], [0.010896697044372123], [0.010896697044372123], [0.010896697044372123], [0.010896697044372123], [0.010896697044372123], [0.010896697044372123], [0.010896697044372123], [0.010896697044372123], [0.010896697044372123], [0.010896697044372123], [0.010896697044372123], [0.010896697044372123], [0.010896697044372123], [0.010896697044372123], [0.010896697044372123], [0.010896697044372123], [0.010896697044372123], [0.010896697044372123], [0.010896697044372123], [0.010896697044372123], [0.010896697044372123], [0.010896697044372123], [0.010896697044372123], [0.010896697044372123], [0.010896697044372123], [0.010896697044372123], [0.010896697044372123], [0.010896697044372123], [0.010896697044372123], [0.010896697044372123], [0.010896697044372123], [0.010896697044372123], [0.010896697044372123], [0.010896697044372123], [0.010896697044372123], [0.010896697044372123], [0.010896697044372123], [0.010896697044372123], [0.010896697044372123], [0.010896697044372123], [0.010896697044372123], [0.010896697044372123], [0.010896697044372123], [0.010896697044372123], [0.010896697044372123], [0.010896697044372123], [0.010896697044372123], [0.010896697044372123], [0.010896697044372123], [0.010896697044372123], [0.010896697044372123], [0.010896697044372123], [0.010896697044372123], [0.010896697044372123], [0.010896697044372123], [0.010896697044372123], [0.010896697044372123], [0.010896697044372123], [0.010896697044372123], [0.010896697044372123], [0.010896697044372123], [0.010896697044372123], [0.010896697044372123], [0.010896697044372123], [0.010896697044372123], [0.010896697044372123], [0.010896697044372123], [0.010896697044372123], [0.010896697044372123], [0.010896697044372123], [0.010896697044372123], [0.010896697044372123], [0.010896697044372123], [0.010896697044372123], [0.010896697044372123], [0.010896697044372123], [0.010896697044372123], [0.010896697044372123], [0.010896697044372123], [0.010896697044372123], [0.010896697044372123], [0.010896697044372123], [0.010896697044372123], [0.010896697044372123], [0.010896697044372123], [0.010896697044372123], [0.010896697044372123], [0.010896697044372123], [0.010896697044372123], [0.010896697044372123], [0.010896697044372123], [0.010896697044372123], [0.010896697044372123], [0.010896697044372123], [0.010896697044372123], [0.010896697044372123], [0.010896697044372123], [0.010896697044372123], [0.010896697044372123], [0.010896697044372123], [0.010896697044372123], [0.010896697044372123], [0.010896697044372123], [0.010896697044372123], [0.010896697044372123], [0.010896697044372123], [0.010896697044372123], [0.010896697044372123], [0.010896697044372123], [0.010896697044372123], [0.010896697044372123], [0.010896697044372123], [0.010896697044372123], [0.010896697044372123], [0.010896697044372123], [0.010896697044372123], [0.010896697044372123], [0.010896697044372123], [0.010896697044372123], [0.010896697044372123], [0.010896697044372123], [0.010896697044372123], [0.010896697044372123], [0.010896697044372123], [0.010896697044372123], [0.010896697044372123], [0.010896697044372123], [0.010896697044372123], [0.010896697044372123], [0.010896697044372123], [0.010896697044372123], [0.010896697044372123], [0.010896697044372123], [0.010896697044372123], [0.010896697044372123], [0.010896697044372123], [0.010896697044372123], [0.010896697044372123], [0.010896697044372123], [0.010896697044372123], [0.010896697044372123], [0.010896697044372123], [0.010896697044372123], [0.010896697044372123], [0.010896697044372123], [0.010896697044372123]], 10 "N":cluster{"N1":dbl, "N2":dbl, "N3":dbl, "N4":dbl}={"N1"=7.00003046875, "N2"=7.00003046875, "N3"=-0.14290789298293544, "N4"=-9.432270749714217e-10} {"N4" format="%#_6p"; "N3" format="%#_6p"; "N2" format="%#_6p"; "N1" format="%#_6p"}, 13 "Index, Wavenames":string[][](table)=[["0", "'time.SA03008H.20180718.000487'\n"], ["1", "'temp.SA03008H.20180718.000487'\n"], ["2", "'B.SA03008H.20180718.000487'\n"], ["3", "'Vsource.SA03008H.20180718.000487'\n"], ["4", "'Lockin0.SA03008H.20180718.000487'\n"], ["5", "'Lockin1.SA03008H.20180718.000487'\n"], ["6", "'Lockin2.SA03008H.20180718.000487'\n"], ["7", "'Lockin3.SA03008H.20180718.000487'\n"], ["8", "'Lockin4.SA03008H.20180718.000487'\n"], ["9", "'Lockin5.SA03008H.20180718.000487'\n"], ["10", "'B_rate.SA03008H.20180718.000487'\n"], ["11", "'DC0.SA03008H.20180718.000487'\n"], ["12", "'DC1.SA03008H.20180718.000487'\n"], ["13", "'DC2.SA03008H.20180718.000487'\n"], ["14", "'DC3.SA03008H.20180718.000487'\n"], ["15", "'DC4.SA03008H.20180718.000487'\n"], ["16", "'DC5.SA03008H.20180718.000487'\n"], ["17", "'DC6.SA03008H.20180718.000487'\n"], ["18", "'DC7.SA03008H.20180718.000487'\n"], ["", ""]], 14 "Comments":string="IGOR\nX// Date: 7/19/2018 6:19 PM\nX// SA03008H\nX// \nX// Source 2 Drain 28 (lockin 1 and 7)\nX// Gohm resistor, sweep BG\nX// \nX// 50mV AC -150mV DC for the IV sweep\nX// \nX// 0 to 15 slowly at 0.25 V step sizes\nX// Stepping B 0-7 @ 1T steps\n\nX// B_Field=7.000000\n\nX// \n\nX// B_Field_Rate=0.400000\n\nX// \n\nX// DAQ_Vbg=15.000000\n\nX// \nX// B= 7.000030\n\n\n\n\n\n\n\n\n\n\n\n\n\n\n\n\n\n\n\n\n\n\n\n\n\n\n\n\n\n\n\n\n\n\n\n\n\n\n\n\nX \nX Display/R 'time.SA03008H.20180718.000487'\nX AppendToGraph 'temp.SA03008H.20180718.000487'\nX AppendToGraph 'B.SA03008H.20180718.000487'\nX AppendToGraph 'Vsource.SA03008H.20180718.000487'\nX AppendToGraph 'Lockin0.SA03008H.20180718.000487'\nX AppendToGraph 'Lockin1.SA03008H.20180718.000487'\nX AppendToGraph 'Lockin2.SA03008H.20180718.000487'\nX AppendToGraph 'Lockin3.SA03008H.20180718.000487'\nX AppendToGraph 'Lockin4.SA03008H.20180718.000487'\nX AppendToGraph 'Lockin5.SA03008H.20180718.000487'\nX AppendToGraph 'B_rate.SA03008H.20180718.000487'\nX AppendToGraph 'DC0.SA03008H.20180718.000487'\nX AppendToGraph 'DC1.SA03008H.20180718.000487'\nX AppendToGraph 'DC2.SA03008H.20180718.000487'\nX AppendToGraph 'DC3.SA03008H.20180718.000487'\nX AppendToGraph 'DC4.SA03008H.20180718.000487'\nX AppendToGraph 'DC5.SA03008H.20180718.000487'\nX AppendToGraph 'DC6.SA03008H.20180718.000487'\nX AppendToGraph 'DC7.SA03008H.20180718.000487'\nX Label bottom \"x label\"\nX Label left \"y label\"\nX ModifyGraph rgb('time.SA03008H.20180718.000487')=(65280,0,0)\nX ModifyGraph rgb('temp.SA03008H.20180718.000487')=(65280,18432,0)\nX ModifyGraph rgb('B.SA03008H.20180718.000487')=(65280,36864,0)\nX ModifyGraph rgb('Vsource.SA03008H.20180718.000487')=(65280,55296,0)\nX ModifyGraph rgb('Lockin0.SA03008H.20180718.000487')=(57344,65280,0)\nX ModifyGraph rgb('Lockin1.SA03008H.20180718.000487')=(37376,65280,0)\nX ModifyGraph rgb('Lockin2.SA03008H.20180718.000487')=(18944,65280,0)\nX ModifyGraph rgb('Lockin3.SA03008H.20180718.000487')=(512,65280,0)\nX ModifyGraph rgb('Lockin4.SA03008H.20180718.000487')=(0,65280,17920)\nX ModifyGraph rgb('Lockin5.SA03008H.20180718.000487')=(0,65280,36352)\nX ModifyGraph rgb('B_rate.SA03008H.20180718.000487')=(0,65280,54784)\nX ModifyGraph rgb('DC0.SA03008H.20180718.000487')=(0,57856,65280)\nX ModifyGraph rgb('DC1.SA03008H.20180718.000487')=(0,39424,65280)\nX ModifyGraph rgb('DC2.SA03008H.20180718.000487')=(0,20992,65280)\nX ModifyGraph rgb('DC3.SA03008H.20180718.000487')=(0,2560,65280)\nX ModifyGraph rgb('DC4.SA03008H.20180718.000487')=(17408,0,65280)\nX ModifyGraph rgb('DC5.SA03008H.20180718.000487')=(35840,0,65280)\nX ModifyGraph rgb('DC6.SA03008H.20180718.000487')=(54272,0,65280)\nX ModifyGraph rgb('DC7.SA03008H.20180718.000487')=(65280,0,58368)\nX Legend/C/N=text0/J \"\\\\s('time.SA03008H.20180718.000487') time\\r\\\\s('temp.SA03008H.20180718.000487') temp\\r\\\\s('B.SA03008H.20180718.000487') B\\r\\\\s('Vsource.SA03008H.20180718.000487') Vsource\\r\\\\s('Lockin0.SA03008H.20180718.000487') Lockin0\\r\\\\s('Lockin1.SA03008H.20180718.000487') Lockin1\\r\\\\s('Lockin2.SA03008H.20180718.000487') Lockin2\\r\\\\s('Lockin3.SA03008H.20180718.000487') Lockin3\\r\\\\s('Lockin4.SA03008H.20180718.000487') Lockin4\\r\\\\s('Lockin5.SA03008H.20180718.000487') Lockin5\\r\\\\s('B_rate.SA03008H.20180718.000487') B_rate\\r\\\\s('DC0.SA03008H.20180718.000487') DC0\\r\\\\s('DC1.SA03008H.20180718.000487') DC1\\r\\\\s('DC2.SA03008H.20180718.000487') DC2\\r\\\\s('DC3.SA03008H.20180718.000487') DC3\\r\\\\s('DC4.SA03008H.20180718.000487') DC4\\r\\\\s('DC5.SA03008H.20180718.000487') DC5\\r\\\\s('DC6.SA03008H.20180718.000487') DC6\\r\\\\s('DC7.SA03008H.20180718.000487') DC7\"\nX ModifyGraph mirror(bottom)=1\nX ModifyGraph width=216\nX ModifyGraph height={Aspect,0.6}\nX ModifyGraph Log(bottom)=0\nX ModifyGraph Log(left)=0\nX \n", 15 "E index vs Field":cluster{i32[], dbl[]}(graph)={[0], [7.00003046875]})   [LabVIEW 2016]
uses:
  <vilib>/Utility/miscctls.llb/LVOffsetAndMultiplierTypeDef.ctl
  <vilib>/Analysis/3filter.llb/Savitzky-Golay Filter (DBL).vi
  <vilib>/Analysis/2dsp.llb/Decimate (single shot, DBL).vi
  <userlib>/LevyLab/LV to ITX/LVtoITX.lvclass
  <vilib>/Analysis/NI_AALPro.lvlib
  <vilib>/Analysis/NI_AALBase.lvlib
panel:
  in  "VRM mode":bool
  in  "Ring":u16(ring) items=["default", "DIFF"]
  in  "decimating factor":i32=1
  in  "decimate files":i32=1
  in  "side points":i32=6
  in  "fit points":dbl=10.0
  in  "dy/dx vs x":bool=TRUE
  in  "Portion of data":cluster{dbl, dbl}(slide)={0.75, 0.25} scale=0.0..1.0
  in  "length 2":i32=2500
  in  "index 2":i32=1072
  out "Ns":T1(array[cluster])=[{"N1"=7.00003046875, "N2"=7.00003046875, "N3"=-0.14290789298293544, "N4"=-9.432270749714217e-10}]
  in  "SE?":bool=TRUE
  in  "D  is time?":bool
  in  "B is time?":bool
  out "time":string[][](table)=[["7/19/2018", "6:19 PM"]]
  in  "Use Folder Index File?":bool
  in  "Generate Folder Index File?":bool
  in  "Ez name":string="Conductance (S)"
  in  "Ey name":string="BY (T)"
  in  "Ex name":string="Vsg (mV)"
  in  "C y name":string="voltage"
  in  "D x name":string="Vsg"
  in  "A y name":string="current"
  in  "B x name":string="Vsg"
  in  "recolor traces?":bool
  in  "Ex":T3={"Offset"=0.0, "Multiplier"=1.0}
  in  "Ey":T3={"Offset"=0.0, "Multiplier"=1.0}
  out "Path":path=path "B:/SketchSET/SA03008H.20180718/51-B+BG_0to15_0.25steps_@0-7T_1step_at.2Hz/SA03008H.20180718.000487.itx"
  out "counter":i32
  in  "pattern":string="*.itx"
  # "A1-A2\nC1-C2\nE-E2"
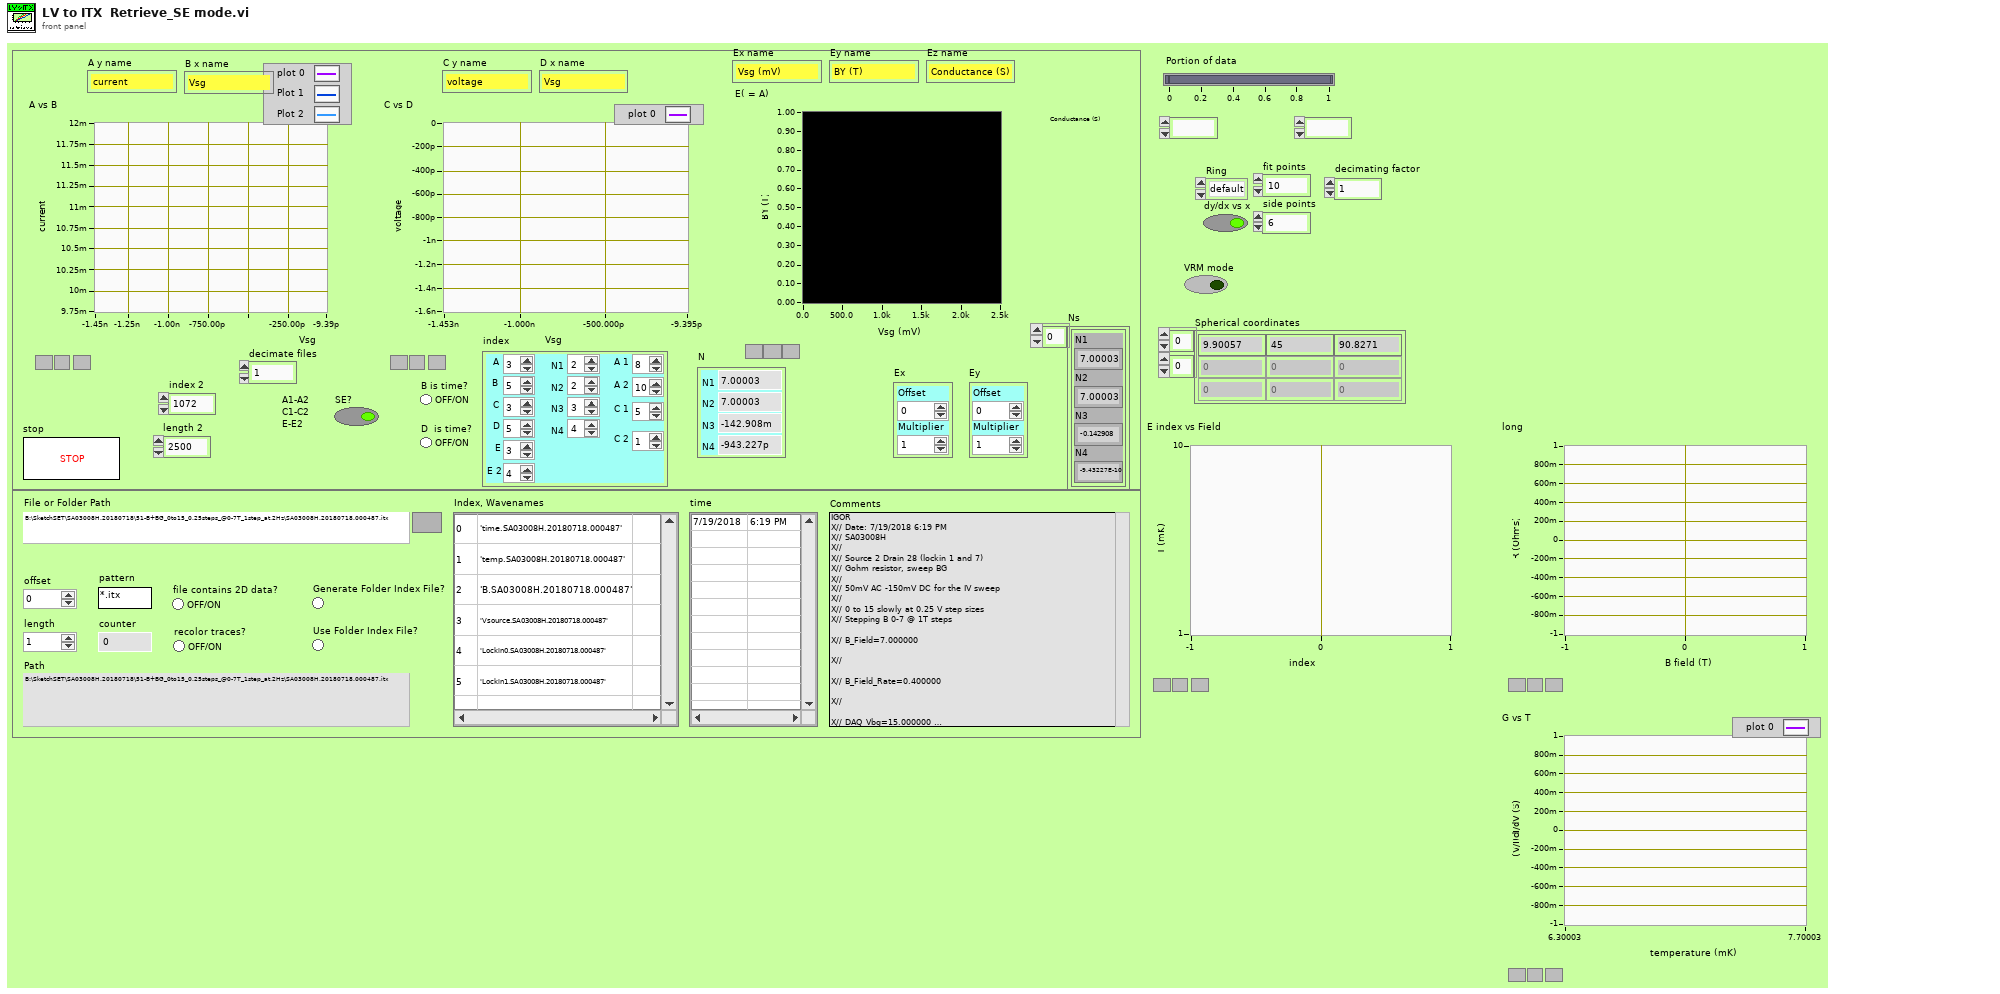
[diagram p1: front panel]
types:
  T1 = cluster{"N1":dbl, "N2":dbl, "N3":dbl, "N4":dbl}[]
  T2 = cluster{"A":i32, "B":i32, "C":i32, "D":i32, "E":i32, "N1":i32, "N2":i32, "N3":i32, "N4":i32, "A 1":i32, "A 2":i32, "C 1":i32, "C 2":i32, "E 2":i32}
  T3 = typedef "LVOffsetAndMultiplierTypeDef.ctl" = cluster{"Offset":dbl, "Multiplier":dbl}
  T4 = cluster{"Decimated Array":dbl[], "Decimated Array":dbl[]}
  T5 = cluster{"Decimated Array":dbl[], "Filtered X":dbl[]}
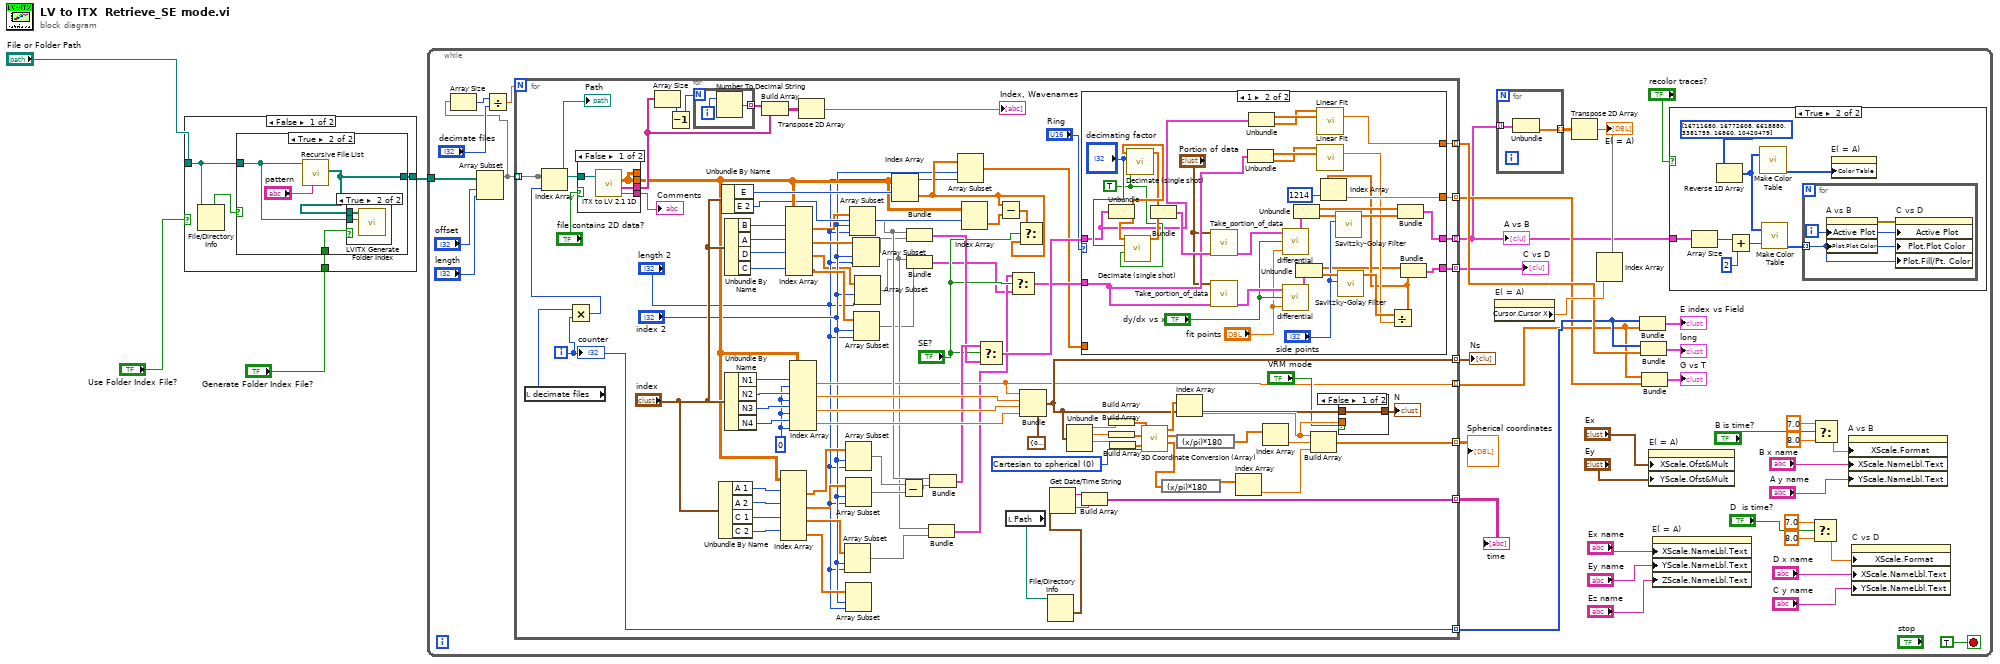
[diagram p0: block diagram]
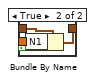
[diagram p3: hidden frame]
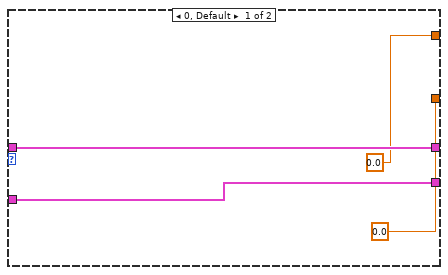
[diagram p4: hidden frame]
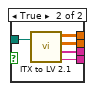
[diagram p5: hidden frame]
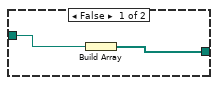
[diagram p6: hidden frame]
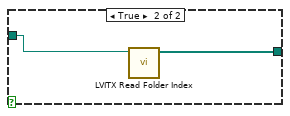
[diagram p8: hidden frame]
diagram:
  n1 = case shown="False" "Use Folder Index File?" {
    tunnel: [w6 w17] -> w2
    tunnel: "File or Folder Path" -> [w8 w18]
    tunnel: "Generate Folder Index File?" -> [w5 _]
    frame False {
      n2 = File/Directory Info(path=w8) -> (directory=w7:bool)  [unwired: 1 in, 6 out]
      n3 = case shown="True" w7 {
        tunnel: [w10 w13] -> w6
        tunnel: w8 -> [w9 w12]
        tunnel: w5 -> [_ w11]
        frame False {
          n4 = Build Array(w9) -> (w10:path[])
        }
        frame True {
          n5 = call <vilib>:"Recursive File List.vi"("pattern"="pattern", "Folder Path"=w12) -> ("All Files in Dir"=w13:path[])  [unwired: 5 in, 4 out]
          n6 = case shown="True" w11 {
            tunnel: w13 -> [_ w16]
            tunnel: w12 -> [_ w15]
            frame False {
            }
            frame True {
              n7 = call <userlib>:"LVITX Generate Folder Index.vi"("File or Folder Path"=w15, "All Files in Dir"=w16) -> ()  [unwired: 10 in]
            }
          }
        }
      }
    }
    frame True {
      n8 = call <userlib>:"LVITX Read Folder Index.vi"("File or Folder Path"=w18) -> ("Array"=w17:path[])  [unwired: 10 in]
    }
  }
  n9 = while {
    tunnel: w2 -> [w36]
    stop <- TRUE stop-if-true
    n10 = Array Subset(array=w36, index="offset", length="length") -> (w32:path[])
    n11 = Array Size(array=w32) -> (size(s)=w35:i32)
    n12 = Divide(x=w35, y="decimate files") -> (x/y=w33:dbl)
    n13 = for {
      N: w33 -> [_]
      tunnel: w32 -> [w164]
      tunnel: [w164] -> _ mode=indexing
      tunnel: [w99] -> w19 mode=indexing
      tunnel: [w98] -> w20 mode=indexing
      tunnel: [w139] -> w50 mode=indexing
      tunnel: [w87] -> w39 mode=indexing
      tunnel: [w97] -> w37 mode=indexing
      tunnel: [w91] -> w29 mode=indexing
      tunnel: [w90] -> w21 mode=indexing
      tunnel: [w84] -> w25 mode=indexing
      tunnel: [w83] -> w24 mode=indexing
      i -> [w84]
      w114 = u16 0 items=["Cartesian to spherical", "spherical to Cartesian", "Cartesian to cylindrical", "cylindrical to Cartesian", "spherical to cylindrical", "cylindrical to spherical"] ("conversion type")
      w137 = 0 ("disabled index (col)")
      n14 = local read "decimate files"() -> (w94:i32)
      n15 = Multiply(x=w94, y=w84) -> (x*y=w95:i32)
      n16 = Index Array(array=w164, index=w95) -> (element=w96:path)
      "Path" <- w96
      n17 = case shown="False" "file contains 2D data?" {
        tunnel: [w213 w216] -> w165
        tunnel: [w211 w217] -> w128
        tunnel: w96 -> [w212 w218]
        tunnel: [w210 w215] -> w157
        tunnel: [w211 w214] -> _
        frame False {
          n18 = call <userlib>:"ITX to LV 2.1 1D.vi"("file (use dialog)"=w212) -> ("array type (2D Dbl)"=w211:dbl[][], "wave names"=w210:string[], "Notes"=w213:string)  [unwired: 2 in]
        }
        frame True {
          n19 = call <userlib>:"ITX to LV 2.1.vi"("file (use dialog)"=w218) -> ("2D array"=w214:dbl[][], "1D arrays"=w217:dbl[][], "wave names"=w215:string[], "Notes"=w216:string)  [unwired: 1 in]
        }
      }
      "Comments" <- w165
      n20 = Array Size(array=w157) -> (size(s)=w160:i32)
      n21 = Decrement(x=w160) -> (x-1=w159:i32)
      n22 = for {
        N: w159 -> [_]
        tunnel: [w208] -> w162 mode=indexing
        i -> [w209]
        n23 = Number To Decimal String(number=w209) -> (decimal integer string=w208:string)  [unwired: 1 in]
      }
      n24 = Unbundle By Name("index") -> ("A 1"=w136:i32, "A 2"=w135:i32, "C 1"=w134:i32, "C 2"=w133:i32)
      n25 = Unbundle By Name("index") -> ("E"=w150:i32, "E 2"=w127:i32)
      n26 = Unbundle By Name("index") -> ("B"=w149:i32, "A"=w148:i32, "D"=w147:i32, "C"=w146:i32)
      n27 = Unbundle By Name("index") -> ("N1"=w151:i32, "N2"=w152:i32, "N3"=w153:i32, "N4"=w154:i32)
      n28 = Build Array(w162, w157) -> (w158:string[][])
      n29 = Index Array(array=w128, index (row) #1=w136, index (row) #2=w135, index (row) #3=w134, index (row) #4=w133) -> (element #1=w119:dbl[], element #2=w117:dbl[], element #3=w116:dbl[], element #4=w115:dbl[])  [unwired: 4 in]
      n30 = Index Array(array=w128, index (row) #1=w149, index (row) #2=w148, index (row) #3=w147, index (row) #4=w146) -> (element #1=w124:dbl[], element #2=w122:dbl[], element #3=w74:dbl[], element #4=w120:dbl[])  [unwired: 4 in]
      n31 = Index Array(array=w128, index (row) #1=w151, index (col) #1=w137, index (row) #2=w152, index (col) #2=w137, index (row) #3=w153, index (col) #3=w137, index (row) #4=w154, index (col) #4=w137) -> (element #1=w83:dbl, element #2=w143:dbl, element #3=w144:dbl, element #4=w156:dbl)
      n32 = Transpose 2D Array(2D array=w158) -> (transposed array=→"Index, Wavenames":string[][])
      n33 = Array Subset(array=w116, index="index 2", length="length 2") -> (w82:dbl[])
      n34 = Array Subset(array=w119, index="index 2", length="length 2") -> (w118:dbl[])
      n35 = Array Subset(array=w117, index="index 2", length="length 2") -> (w89:dbl[])
      n36 = Array Subset(array=w115, index="index 2", length="length 2") -> ()  [unwired: 1 out]
      n37 = Array Subset(array=w124, index="index 2", length="length 2") -> (w123:dbl[])
      n38 = Array Subset(array=w122, index="index 2", length="length 2") -> (w121:dbl[])
      n39 = Array Subset(array=w120, index="index 2", length="length 2") -> (w73:dbl[])
      n40 = Array Subset(array=w74, index="index 2", length="length 2") -> (w75:dbl[])
      n41 = Index Array(array=w128, index (row)=w150) -> (element=w79:dbl[])  [unwired: 1 in]
      n42 = Subtract(x=w118, y=w89) -> (x-y=w132:dbl[])
      n43 = Bundle(w123, w121) -> (w130:cluster{dbl[], dbl[]})  [unwired: 1 in]
      n44 = Bundle(w75, w73) -> (w80:cluster{dbl[], dbl[]})  [unwired: 1 in]
      n45 = Bundle(w75, w82) -> (w81:cluster{dbl[], dbl[]})  [unwired: 1 in]
      n46 = Bundle(w123, w132) -> (w131:cluster{dbl[], dbl[]})  [unwired: 1 in]
      n47 = Array Subset(array=w79, index="index 2", length="length 2") -> (w76:dbl[])
      n48 = Index Array(array=w128, index (row)=w127) -> (element=w126:dbl[])  [unwired: 1 in]
      n49 = Select(t=w131, s="SE?", f=w130) -> (s? t:f=w101:cluster{dbl[], dbl[]})
      n50 = Subtract(x=w79, y=w126) -> (x-y=w125:dbl[])
      n51 = local read "Path"() -> (w145:path)
      n52 = Select(t=w81, s="SE?", f=w80) -> (s? t:f=w100:cluster{dbl[], dbl[]})
      n53 = Select(t=w125, s="SE?", f=w79) -> ()  [unwired: 1 out]
      n54 = Bundle(cluster=cluster{"N1":dbl, "N2":dbl, "N3":dbl, "N4":dbl} {"N1"=0.0, "N2"=0.0, "N3"=0.0, "N4"=0.0}, "N1"=w83, "N2"=w143, "N3"=w144, "N4"=w156) -> (w87:cluster{"N1":dbl, "N2":dbl, "N3":dbl, "N4":dbl})
      n55 = File/Directory Info(path=w145) -> (last mod=w142:timestamp)  [unwired: 1 in, 6 out]
      n56 = Get Date/Time String(seconds (now)=w142) -> (date string=w141:string, time string=w140:string)  [unwired: 2 in]
      n57 = Unbundle(w87) -> ("N1"=w93:dbl, "N2"=w113:dbl, "N3"=w110:dbl)  [unwired: 1 out]
      n58 = case shown="1" "Ring" {
        tunnel: w101 -> [w173 w191]
        tunnel: w100 -> [w172 w180]
        tunnel: [w173 w176] -> w99
        tunnel: [w172 w175] -> w98
        tunnel: [0.0 w188] -> w91
        tunnel: [0.0 w185] -> w90
        tunnel: w76 -> [_ _]
        frame 0, Default {
        }
        frame 1 {
          w192 = TRUE ("averaging")
          n59 = Unbundle(w191) -> (w197:dbl[], w195:dbl[])
          n60 = call-poly <vilib>:"Decimate (single shot).vi"("averaging"=w192, "decimating factor"="decimating factor", "X"=w195) -> ("Decimated Array"=w194:dbl[])  [unwired: 7 in, 1 out]
          n61 = call-poly <vilib>:"Decimate (single shot).vi"("averaging"=w192, "decimating factor"="decimating factor", "X"=w197) -> ("Decimated Array"=w196:dbl[])  [unwired: 7 in, 1 out]
          n62 = Bundle("Decimated Array"=w196, "Decimated Array"=w194) -> (w198:T4)  [unwired: 1 in]
          n63 = call <userlib>:"Take_portion_of_data.vi"("input IV"=w198, "Slide"="Portion of data") -> ("Output IV"=w206:cluster{dbl[], dbl[]})  [unwired: 5 in]
          n64 = call <userlib>:"Take_portion_of_data.vi"("input IV"=w180, "Slide"="Portion of data") -> ("Output IV"=w207:cluster{dbl[], dbl[]})  [unwired: 5 in]
          n65 = Unbundle(w180) -> (w189:dbl[], w184:dbl[])
          n66 = Unbundle(w191) -> (w190:dbl[], w187:dbl[])
          n67 = call <userlib>:"differential.vi"("Numeric"="fit points", "dy/dx vs x"="dy/dx vs x", "A vs B 2"=w206) -> ("A vs B 3"=w202:T4)  [unwired: 1 in]
          n68 = call <userlib>:"differential.vi"("Numeric"="fit points", "dy/dx vs x"="dy/dx vs x", "A vs B 2"=w207) -> ("A vs B 3"=w200:T4)  [unwired: 1 in]
          n69 = Unbundle(w202) -> ("Decimated Array"=w205:dbl[], "Decimated Array"=w203:dbl[])
          n70 = Unbundle(w200) -> ("Decimated Array"=w174:dbl[], "Decimated Array"=w201:dbl[])
          n71 = call <vilib>:"Linear Fit.vi"("Y"=w187, "X"=w190) -> ("slope"=w188:dbl)  [unwired: 9 in, 4 out]
          n72 = call <vilib>:"Linear Fit.vi"("Y"=w184, "X"=w189) -> ("slope"=w182:dbl)  [unwired: 9 in, 4 out]
          n73 = call-poly <vilib>:"Savitzky-Golay Filter.vi"("side points"="side points", "X"=w203) -> ("Filtered X"=w204:dbl[])  [unwired: 8 in, 1 out]
          n74 = call-poly <vilib>:"Savitzky-Golay Filter.vi"("side points"="side points", "X"=w201) -> ("Filtered X"=w183:dbl[])  [unwired: 8 in, 1 out]
          n75 = Divide(x=w183, y=w182) -> (x/y=w181:dbl[])
          n76 = Index Array(array=w181, index=1214) -> (element=w185:dbl)
          n77 = Bundle("Decimated Array"=w205, "Filtered X"=w204) -> (w176:T5)  [unwired: 1 in]
          n78 = Bundle("Decimated Array"=w174, w181) -> (w175:cluster{"Decimated Array":dbl[], dbl[]})  [unwired: 1 in]
        }
      }
      n79 = Build Array(w141, w140) -> (w139:string[])
      n80 = Build Array(w93) -> (w112:dbl[])
      n81 = Build Array(w113) -> (w111:dbl[])
      n82 = Build Array(w110) -> (w109:dbl[])
      n83 = call <vilib>:"3D Coordinate Conversion (Array).vi"("conversion type"=w114, "Axis 3"=w109, "Axis 2"=w111, "Axis 1"=w112) -> ("Axis 3 Out"=w107:dbl[], "Axis 2 Out"=w108:dbl[], "Axis 1 Out"=w106:dbl[])  [unwired: 4 in, 1 out]
      n84 = expression code="(x/pi)*180" ("degrees to radians")(w107) -> (w104:dbl[])
      n85 = Index Array(array=w106) -> (element=w88:dbl)  [unwired: 1 in]
      n86 = expression code="(x/pi)*180" ("degrees to radians")(w108) -> (w105:dbl[])
      n87 = Index Array(array=w104) -> (element=w102:dbl)  [unwired: 1 in]
      n88 = Index Array(array=w105) -> (element=w103:dbl)  [unwired: 1 in]
      n89 = Build Array(w88, w103, w102) -> (w97:dbl[])
      n90 = case shown="False" "VRM mode" {
        tunnel: w88 -> [_ w169]
        tunnel: w87 -> [w166 w168]
        tunnel: [w166 w167] -> w86
        frame False {
        }
        frame True {
          n91 = Bundle By Name(cluster=w168, "N1"=w169) -> (w167:cluster{"N1":dbl, "N2":dbl, "N3":dbl, "N4":dbl})
        }
      }
      "N" <- w86
      "counter" <- w84
    }
    "time" <- w50
    "Ns" <- w39
    "Spherical coordinates" <- w37
    "A vs B" <- w19
    "C vs D" <- w20
    n92 = property on="E( = A)" class="IntGraph (strict)"() -> ("Cursor.Cursor X"=w30:dbl)  [unwired: 2 in, 2 out]
    n93 = for {
      tunnel: [w60] -> _ mode=indexing
      tunnel: [w61] -> w38 mode=indexing
      tunnel: w19 -> [w60] mode=indexing
      n94 = Unbundle(w60) -> ("Filtered X"=w61:dbl[])  [unwired: 1 out]
    }
    n95 = Transpose 2D Array(2D array=w38) -> (transposed array=w22:dbl[][])
    "E( = A)" <- w22
    n96 = Index Array(array=w22, index (row)=w30) -> ()  [unwired: 1 in, 1 out]
    n97 = Bundle(w25, w24) -> (→"E index vs Field":cluster{i32[], dbl[]})  [unwired: 1 in]
    n98 = Bundle(w25, w29) -> (→"long":cluster{i32[], dbl[]})  [unwired: 1 in]
    n99 = Bundle(w24, w21) -> (→"G vs T":cluster{dbl[], dbl[]})  [unwired: 1 in]
    n100 = property on="E( = A)" class="IntGraph (strict)"("XScale.Ofst&Mult"="Ex", "YScale.Ofst&Mult"="Ey") -> ()  [unwired: 2 in, 2 out]
    n101 = property on="E( = A)" class="IntGraph (strict)"("XScale.NameLbl.Text"="Ex name", "YScale.NameLbl.Text"="Ey name", "ZScale.NameLbl.Text"="Ez name") -> ()  [unwired: 2 in, 2 out]
    n102 = case shown="True" "recolor traces?" {
      tunnel: w19 -> [_ w64]
      frame False {
      }
      frame True {
        n103 = Array Size(array=w64) -> (size(s)=w65:i32)
        n104 = Reverse 1D Array(array=u32[] [16711680, 16772608, 6618880, 3381759, 16860, 10420479] ("color scale")) -> (reversed array=w63:u32[])
        n105 = Add(x=w65, y=2 ("x")) -> (x+y=w69:i32)
        n106 = call <userlib>:"Make Color Table.vi"("Array"=w63) -> ("Color Tbl"=w67:u32[])  [unwired: 1 in, 3 out]
        n107 = call <userlib>:"Make Color Table.vi"("Array"=w63, "Size/3"=w69) -> ("Color Tbl"=w66:u32[])  [unwired: 3 out]
        n108 = for {
          tunnel: w66 -> [w70] mode=indexing
          i -> [w71]
          n109 = property on="A vs B" class="XYGraph (strict)"("Active Plot"=w71, "Plot.Plot Color"=w70) -> (error out=w72:errorcluster)  [unwired: 2 in, 1 out]
          n110 = property on="C vs D" class="XYGraph (strict)"(error in=w72, "Active Plot"=w71, "Plot.Plot Color"=w70, "Plot.Fill/Pt. Color"=w70) -> ()  [unwired: 1 in, 2 out]
        }
        n111 = property on="E( = A)" class="IntGraph (strict)"("Color Table"=w67) -> ()  [unwired: 2 in, 2 out]
      }
    }
    n112 = Select(t=7.0, s="D  is time?", f=8.0) -> (s? t:f=w44:dbl)
    n113 = Select(t=7.0, s="B is time?", f=8.0) -> (s? t:f=w45:dbl)
    n114 = property on="A vs B" class="XYGraph (strict)"("XScale.Format"=w45, "XScale.NameLbl.Text"="B x name", "YScale.NameLbl.Text"="A y name") -> ()  [unwired: 2 in, 2 out]
    n115 = property on="C vs D" class="XYGraph (strict)"("XScale.Format"=w44, "XScale.NameLbl.Text"="D x name", "YScale.NameLbl.Text"="C y name") -> ()  [unwired: 2 in, 2 out]
  }
